vi "numeric_addition.vi"() -> ()   [LabVIEW 2019]
panel:
  out "Numeric 2":dbl
  in  "Numeric":dbl
  # "add 200 to the Numeric and output to Numeric 2"
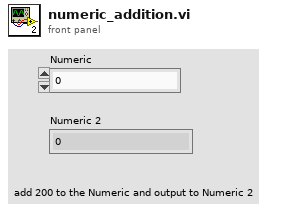
[diagram p1: front panel]
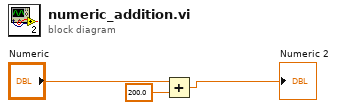
[diagram p0: block diagram]
diagram:
  n1 = Add(x="Numeric", y=200.0) -> (x+y=→"Numeric 2":dbl)
